vi "Periodic Tasks.vi"(8 "error in":errorcluster) -> ()   [LabVIEW 2020]
doc: "This VI runs in parallel to other tasks. It can contain as many user-defined periodic loops as you need. These can carry out PID or other sorts of timed response."
uses:
  <vilib>/Rock Robotics/WPI/ThirdParty/Phoenix-LabVIEW/Motor Controller/Controls/CTRE_Phoenix_MotorControl_ControlMode.ctl
  AutonBoolean.vi
panel:
  # "WHEELS:\nINTAKE 2 GEARS OUT\nSHOOT 2 GEARS IN"
  # "ALL POSITIVE .005"
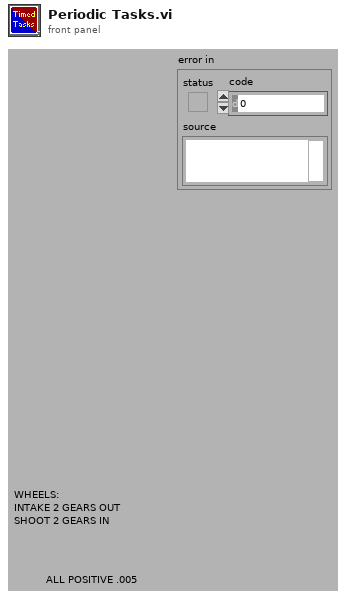
[diagram p1: front panel]
types:
  T1 = cluster{"A":bool, "B":bool, "X":bool, "Y":bool, "Left Bumper":bool, "Right Bumper":bool, "View Button":bool, "Menu Button":bool, "Left Joystick Press":bool, "Right Joystick Press":bool, "Left Thumbpad X Axis":dbl, "Left Thumbpad Y Axis":dbl, "Left Trigger":dbl, "Right Trigger":dbl, "Right Thumbpad X Axis":dbl, "Right Thumbpad Y Axis":dbl, "Driver - Trigger":bool, "Driver - Middle Thumb":bool, "Driver - Left Thumb":bool, "Driver - Right Thumb":bool, "Driver - Left Top Left ":bool, "Driver - Left Top Middle":bool, "Driver - Left Top Right":bool, "Driver - Left Bottom Right":bool, "Driver - Left Bottom Middle":bool, "Driver - Left Bottom Left":bool, "Driver - Right Top Right":bool, "Driver - Right Top Middle":bool, "Driver - Right Top Left":bool, "Driver - Right Bottom Left":bool, "Driver - Right Bottom Middle":bool, "Driver - Right Bottom Right":bool, "Driver - X Axis":dbl, "Driver - Y Axis":dbl, "Driver - Z Axis":dbl}
  T2 = typedef "WPI_MotorControlDeviceRef.ctl" = cluster{"DeviceStatus":errorcluster, "Type":T3, "PWM":cluster{"PWM Channel":T4, "DeadBand":T5}, "CAN":cluster{"Device Number":u8, "SetOutput VI Ref":variant, "GetOutput VI Ref":variant, "Enable VI Ref":variant, "Disable VI Ref":variant, "Data":variant}, "Invert":bool, "DIO PWM":cluster{"PWM \"Enable\" Channel":T4, "DIOChannel":T6, "PWM Rate":dbl}}
  T3 = typedef "WPI_MotorControlType.ctl" = enum16{"PWM", "CAN", "DIO PWM"}
  T4 = typedef "FPGA_DIOPWMChannel.ctl" = enum8{"PWM 0", "PWM 1", "PWM 2", "PWM 3", "PWM 4", "PWM 5", "PWM 6", "PWM 7", "PWM 8", "PWM 9", "PWM MXP 0", "PWM MXP 1", "PWM MXP 2", "PWM MXP 3", "PWM MXP 4", "PWM MXP 5", "PWM MXP 6", "PWM MXP 7", "PWM MXP 8", "PWM MXP 9", "Invalid"}
  T5 = typedef "WPI_PWMDeadband.ctl" = cluster{"Name":string, "maxPositivePwm":i32, "minPositivePwm":i32, "centerPwm":i32, "maxNegativePwm":i32, "minNegativePwm":i32, "angularRange":u16}
  T6 = typedef "FPGA_DIOChannel.ctl" = enum8{"DIO 0", "DIO 1", "DIO 2", "DIO 3", "DIO 4", "DIO 5", "DIO 6", "DIO 7", "DIO 8", "DIO 9", "DIO MXP 0", "DIO MXP 1", "DIO MXP 2", "DIO MXP 3", "DIO MXP 4", "DIO MXP 5", "DIO MXP 6", "DIO MXP 7", "DIO MXP 8", "DIO MXP 9", "DIO MXP 10", "DIO MXP 11", "DIO MXP 12", "DIO MXP 13", "DIO MXP 14", "DIO MXP 15", "SPI Port CS1", "SPI Port CS2", "SPI Port CS3", "SPI Port MISO", "SPI Port MOSI", "Invalid"}
  T7 = typedef "CTRE_Phoenix_MotorControl_ControlMode.ctl" = u16
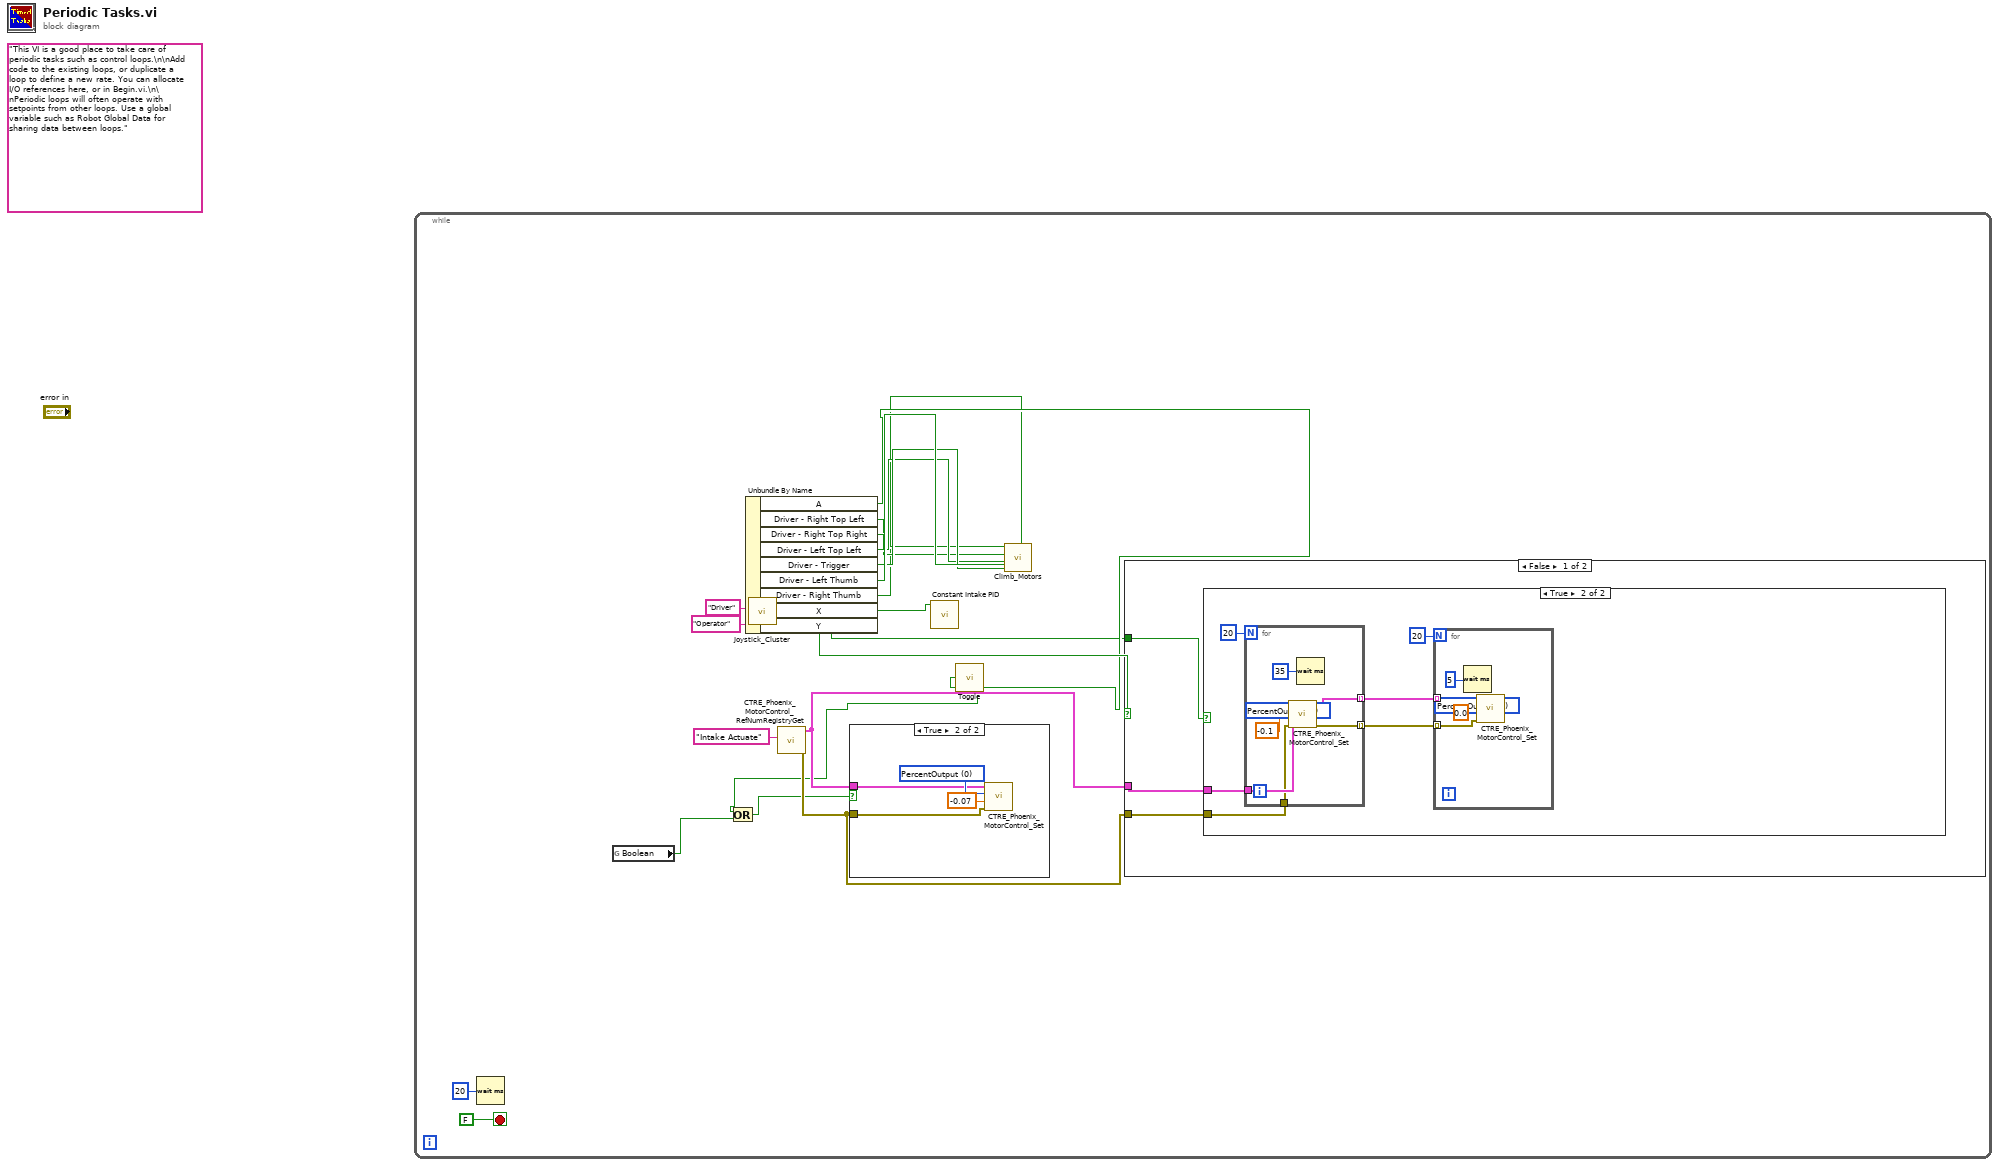
[diagram p0: block diagram]
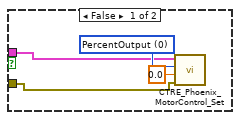
[diagram p2: hidden frame]
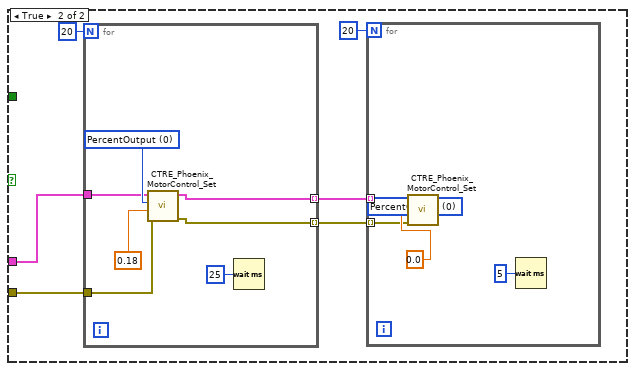
[diagram p4: hidden frame]
diagram:
  (unwired) "This VI is a good place to take care of periodic tasks such as control loops.\n\nAdd code to the existing loops, or duplicate a loop to define a new rate. You can allocate I/O references here, or in Begin.vi.\n\nPeriodic loops will often operate with setpoints from other loops. Use a global variable such as Robot Global Data for sharing data between loops."
  n1 = while {
    stop <- FALSE stop-if-true
    n2 = Wait (ms)(milliseconds to wait=u32 20) -> ()  [unwired: 1 out]
    n3 = global read "AutonBoolean.vi" "Boolean"() -> (w3:bool)
    n4 = call "Joystick_Cluster.vi"("Xbox"="Operator", "Thrustmaster"="Driver") -> ("Joystick Output"=w16:T1)  [unwired: 9 in]
    n5 = Unbundle By Name(w16) -> ("A"=w6:bool, "Driver - Right Top Left"=w9:bool, "Driver - Right Top Right"=w10:bool, "Driver - Left Top Left"=w11:bool, "Driver - Trigger"=w12:bool, "Driver - Left Thumb"=w13:bool, "Driver - Right Thumb"=w2:bool, "X"=w1:bool, "Y"=w15:bool)
    n6 = call <vilib>:"CTRE_Phoenix_MotorControl_RefNumRegistryGet.vi"("refnum name"="Intake Actuate") -> ("error out"=w7:errorcluster, "PhoenixMotorControlDevRef"=w8:T2)  [unwired: 9 in]
    n7 = call "Constant Intake PID.vi"("Boolean"=w1) -> ()  [unwired: 11 in]
    n8 = call "Toggle.vi"("Boolean"=w6) -> ("Boolean Out"=w5:bool)
    n9 = Or(x=w5, y=w3) -> (x .or. y?=w4:bool)
    n10 = case shown="True" w4 {
      tunnel: w8 -> [w22 w26]
      tunnel: w7 -> [w21 w25]
      frame False {
        w23 = T7 0 items=["PercentOutput"=0, "Position"=1, "Velocity"=2, "Current"=3, "Follower"=5, "MotionProfile"=6, "MotionMagic"=7, "MotionProfileArc"=10, "Disabled"=15] ("Control Mode")
        n11 = call <vilib>:"CTRE_Phoenix_MotorControl_Set.vi"("error in (no error)"=w21, "Output"=0.0, "Control Mode"=w23, "PhoenixMotorControlDevRef"=w22) -> ()  [unwired: 6 in, 2 out]
      }
      frame True {
        w27 = T7 0 items=["PercentOutput"=0, "Position"=1, "Velocity"=2, "Current"=3, "Follower"=5, "MotionProfile"=6, "MotionMagic"=7, "MotionProfileArc"=10, "Disabled"=15] ("Control Mode")
        n12 = call <vilib>:"CTRE_Phoenix_MotorControl_Set.vi"("error in (no error)"=w25, "Output"=-0.07, "Control Mode"=w27, "PhoenixMotorControlDevRef"=w26) -> ()  [unwired: 6 in, 2 out]
      }
    }
    n13 = call "Climb_Motors.vi"("Driver - Right Thumb"=w2, "Driver - Left Thumb"=w13, "Driver - Trigger"=w12, "Driver - Left Top left"=w11, "Driver - Right Top Right"=w10, "Driver - Right Top Left"=w9) -> ()  [unwired: 6 in]
    n14 = case shown="False" w15 {
      tunnel: w1 -> [w31 _]
      tunnel: w8 -> [w30 w51]
      tunnel: w7 -> [w29 w50]
      frame False {
        n15 = case shown="True" w31 {
          tunnel: w30 -> [_ w33]
          tunnel: w29 -> [_ w32]
          frame False {
          }
          frame True {
            n16 = for {
              N: 20 -> [_]
              tunnel: [w49] -> w37 mode=indexing
              tunnel: [w48] -> w36 mode=indexing
              tunnel: w33 -> [w44]
              tunnel: w32 -> [w43]
              w46 = T7 0 items=["PercentOutput"=0, "Position"=1, "Velocity"=2, "Current"=3, "Follower"=5, "MotionProfile"=6, "MotionMagic"=7, "MotionProfileArc"=10, "Disabled"=15] ("Control Mode")
              n17 = call <vilib>:"CTRE_Phoenix_MotorControl_Set.vi"("error in (no error)"=w43, "Output"=-0.1, "Control Mode"=w46, "PhoenixMotorControlDevRef"=w44) -> ("error out"=w48:errorcluster, "PhoenixMotorControlDevRef"=w49:T2)  [unwired: 6 in]
              n18 = Wait (ms)(milliseconds to wait=u32 35) -> ()  [unwired: 1 out]
            }
            n19 = for {
              N: 20 -> [_]
              tunnel: w37 -> [w42] mode=indexing
              tunnel: w36 -> [w41] mode=indexing
              w39 = T7 0 items=["PercentOutput"=0, "Position"=1, "Velocity"=2, "Current"=3, "Follower"=5, "MotionProfile"=6, "MotionMagic"=7, "MotionProfileArc"=10, "Disabled"=15] ("Control Mode")
              n20 = Wait (ms)(milliseconds to wait=u32 5) -> ()  [unwired: 1 out]
              n21 = call <vilib>:"CTRE_Phoenix_MotorControl_Set.vi"("error in (no error)"=w41, "Output"=0.0, "Control Mode"=w39, "PhoenixMotorControlDevRef"=w42) -> ()  [unwired: 6 in, 2 out]
            }
          }
        }
      }
      frame True {
        n22 = for {
          N: 20 -> [_]
          tunnel: [w64] -> w54 mode=indexing
          tunnel: [w63] -> w53 mode=indexing
          tunnel: w51 -> [w62]
          tunnel: w50 -> [w61]
          w65 = T7 0 items=["PercentOutput"=0, "Position"=1, "Velocity"=2, "Current"=3, "Follower"=5, "MotionProfile"=6, "MotionMagic"=7, "MotionProfileArc"=10, "Disabled"=15] ("Control Mode")
          n23 = call <vilib>:"CTRE_Phoenix_MotorControl_Set.vi"("error in (no error)"=w61, "Output"=0.18, "Control Mode"=w65, "PhoenixMotorControlDevRef"=w62) -> ("error out"=w63:errorcluster, "PhoenixMotorControlDevRef"=w64:T2)  [unwired: 6 in]
          n24 = Wait (ms)(milliseconds to wait=u32 25) -> ()  [unwired: 1 out]
        }
        n25 = for {
          N: 20 -> [_]
          tunnel: w54 -> [w57] mode=indexing
          tunnel: w53 -> [w56] mode=indexing
          w58 = T7 0 items=["PercentOutput"=0, "Position"=1, "Velocity"=2, "Current"=3, "Follower"=5, "MotionProfile"=6, "MotionMagic"=7, "MotionProfileArc"=10, "Disabled"=15] ("Control Mode")
          n26 = call <vilib>:"CTRE_Phoenix_MotorControl_Set.vi"("error in (no error)"=w56, "Output"=0.0, "Control Mode"=w58, "PhoenixMotorControlDevRef"=w57) -> ()  [unwired: 6 in, 2 out]
          n27 = Wait (ms)(milliseconds to wait=u32 5) -> ()  [unwired: 1 out]
        }
      }
    }
  }
